vi "Benchmark FIFO delay_sim.vi"() -> ()   [LabVIEW 2011]
uses:
  <vilib>/Platform/TimedLoop/XDataNode/timing_clust.ctl
  <vilib>/Platform/TimedLoop/XDataNode/nitl_modes.ctl
  <vilib>/Platform/TimedLoop/XDataNode/wakeup.ctl
  <vilib>/rvi/DataTransferAndStorage/Container/Common/niFpgaContainerExecOnDevCompGetState.vi
  <vilib>/rvi/FIFO/Fifo_Resource/nirvififoEmulationSetSize.vi
  <vilib>/rvi/DataTransferAndStorage/Container/Common/niFpgaContainerGetUniqueNameForEmu.vi
  <vilib>/rvi/interface/RandomDataEmulation/nirviRandomDataFPGAFIFO.vi
  <vilib>/rvi/interface/RandomDataEmulation/niFpgaRandomDataHandleErrors.vi
  <vilib>/rvi/eio/common/nirviEmuReportErrorAndStop.vi
  <vilib>/Platform/TimedLoop/XDataNode/XDataNode.xnode
  <vilib>/rvi/FXPMathLib/basic elements/FxpDiscreteDelay/XNode/nifxpmath_DiscreteDelay.xnode
  <vilib>/rvi/DataTransferAndStorage/Container/XNode/niFpgaContainer.xnode
  <vilib>/rvi/FIFO/Fifo_Resource/niFpgaFifoEmulationRefIn.vi
  <vilib>/Platform/TimedLoop/XDataNode/XDNodeRunTimeDep.lvlib
panel:
  out "Element 4":i16[](array[numeric])
  out "Element 3":i16[](array[numeric])
  out "Write[N-7]":bool
  in  "Element 2":i16[](array[numeric])=[0, 0, 0, 0, 0, 0, 0, 0]
  out "Write[N-6]":bool
  out "Write[N-5]":bool
  out "Write[N-4]":bool
  out "Write[N-3]":bool
  out "Write[N-2]":bool
  out "Write[N-1]":bool
  out "Write[N]":bool
  in  "Write":bool
  # "200M -> N-5"
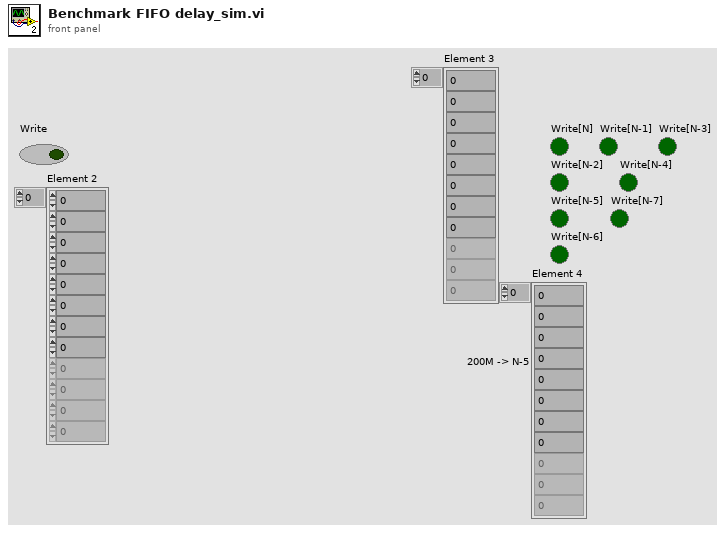
[diagram p1: front panel]
types:
  T1 = typedef "XDNodeRunTimeDep.lvlib/timing_clust.ctl" = cluster{"Expected End [f-1]":u64, "Actual End [f-1]":u64, "Finished Late? [f-1]":bool, "Expected End [i-1]":u64, "Actual End [i-1]":u64, "Finished Late? [i-1]":bool, "Expected Start [i]":u64, "Actual Start [i]":u64, "Expected Start [f]":u64, "Actual Start [f]":u64, "Source Name":string, "Structure Name":string, "Period":i64, "Deadline":i64, "Offset":i64, "Start":i64, "Priority":i32, "Timeout":i32, "Mode":T2, "Wakeup Reason":T3, "Error":errorcluster, "Source Type":string, "Secondary Source Type":string, "Global End Time":u64, "Global Start Time":u64, "Frame Duration":u64, "Iteration Duration":u64, "Assigned CPU":i32, "I/O Scan Engine Mode":u32}
  T2 = typedef "XDNodeRunTimeDep.lvlib/nitl_modes.ctl" = enum32{"No Change", "Process missed periods, maintain original phase", "Discard missed periods, maintain original phase", "Process missed periods, ignore original phase", "Discard missed periods, ignore original phase"}
  T3 = typedef "XDNodeRunTimeDep.lvlib/wakeup.ctl" = enum32{"Normal", "Aborted", "Asynchronous wakeup", "Timing source error", "Timed loop error", "Timeout"}
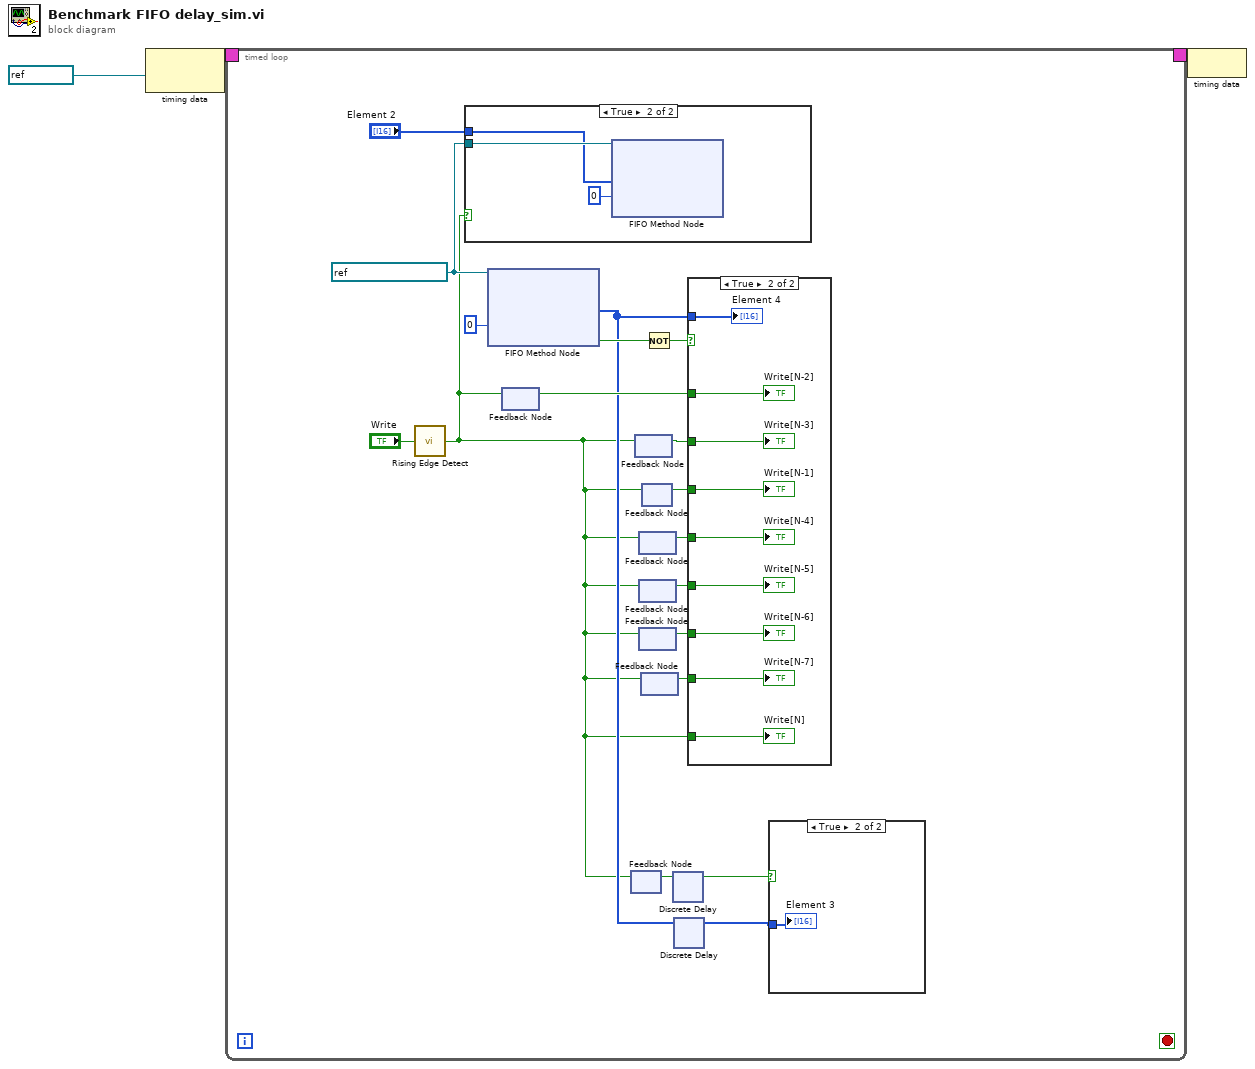
[diagram p0: block diagram]
diagram:
  n1 = node-c288(refnum<k21> "80MHz" ("Source Name")) -> (w3:T1)
  n2 = timed-loop {
    timing: w3 -> [_]
    timing-out: [_] -> w2
    stop <- _ stop-if-true
    w21 = refnum<k21> "HistoryFIFOU128" ("FIFO Out")
    n3 = call <userlib>:"Rising Edge Detect.vi"("signal"="Write") -> ("edge detected"=w4:bool)  [unwired: 14 in]
    n4 = case shown="True" w4 {
      tunnel: w21 -> [_ w34]
      tunnel: "Element 2" -> [_ w32]
      frame False {
      }
      frame True {
        n5 = xnode ("FIFO Method Node")("Element"=w32, "Timeout"=0, "FIFO In"=w34) -> ()  [unwired: 2 out]
      }
    }
    n6 = xnode ("FIFO Method Node")("Timeout"=0, "FIFO In"=w21) -> ("Element"=w6:i16[], "Timed Out?"=w19:bool)  [unwired: 1 out]
    n7 = feedback #1() -> (w14:bool)  [unwired: 1 in]
    n8 = feedback-in #1(w4) -> ()
    n9 = feedback #2() -> (w5:bool)  [unwired: 1 in]
    n10 = feedback-in #2(w4) -> ()
    n11 = feedback #3() -> (w15:bool)  [unwired: 1 in]
    n12 = feedback-in #3(w4) -> ()
    n13 = feedback #4() -> (w16:bool)  [unwired: 1 in]
    n14 = feedback-in #4(w4) -> ()
    n15 = feedback #5() -> (w10:bool)  [unwired: 1 in]
    n16 = feedback-in #5(w4) -> ()
    n17 = feedback #6() -> (w13:bool)  [unwired: 1 in]
    n18 = feedback-in #6(w4) -> ()
    n19 = feedback #7() -> (w11:bool)  [unwired: 1 in]
    n20 = feedback-in #7(w4) -> ()
    n21 = feedback #8() -> (w9:bool)  [unwired: 1 in]
    n22 = feedback-in #8(w4) -> ()
    n23 = Not(x=w19) -> (.not. x?=w17:bool)
    n24 = xnode "Discrete Delay"("D"=w5) -> ("Q"=w8:bool)
    n25 = xnode "Discrete Delay"("D"=w6) -> ("Q"=w7:i16[])
    n26 = case shown="True" w17 {
      tunnel: w4 -> [_ w31]
      tunnel: w9 -> [_ w30]
      tunnel: w16 -> [_ w27]
      tunnel: w15 -> [_ w28]
      tunnel: w14 -> [_ w29]
      tunnel: w10 -> [_ w26]
      tunnel: w13 -> [_ w25]
      tunnel: w11 -> [_ w24]
      tunnel: w6 -> [_ w23]
      frame False {
      }
      frame True {
        "Write[N]" <- w31
        "Write[N-1]" <- w30
        "Write[N-2]" <- w29
        "Write[N-3]" <- w28
        "Write[N-4]" <- w27
        "Write[N-5]" <- w26
        "Write[N-6]" <- w25
        "Write[N-7]" <- w24
        "Element 4" <- w23
      }
    }
    n27 = case shown="True" w8 {
      tunnel: w7 -> [_ w22]
      frame False {
      }
      frame True {
        "Element 3" <- w22
      }
    }
  }
  n28 = node-c288(w2) -> ()
